vi "Main.vi"(11 "Module Admin":refnum<class "Delacor_lib_QMH_Module Admin.lvclass">) -> ()   [LabVIEW 2023, in "Adjust FP VIs.lvlib"]
doc: "This template is based off of the Queued Message Handler design pattern and the Queued Message Handler project template that ships with LabVIEW.\n\nThe main difference is that the queue is private to this module and communication between modules is performed via Broadcast and Request events.\n\nRequest events are wrapped in public API methods and are handled in the Event Handling Loop (EHL) of this VI. Any module can register for Broadcast events sent by this module. The EHL generates messages based on user interface actions.\n\nThe Message Handling Loop (MHL) processes messages generated by the EHL, or by other messages. The messages are string values, so new messages can be added easily to the Message Cases case structure in the MHL. Each message cluster can also provide an optional value for Message Data, which is a variant that can be converted to whatever message-specific data is required.\n_____\nBased on DQMH Dev Tools: Project Template 7.1.2.1547."
uses:
  Adjust FP VIs.lvlib
  <vilib>/Delacor/Delacor QMH/Libraries/Module Admin_class/Delacor_lib_QMH_Module Admin.lvclass
  Module Data--cluster.ctl
  Stop Argument--cluster.ctl
  <vilib>/Delacor/Delacor QMH/Libraries/Message Queue_class/Delacor_lib_QMH_Message Queue.lvclass/Delacor_lib_QMH_Message Queue.ctl
  <vilib>/Delacor/Delacor QMH/Libraries/Module Admin_class/Delacor_lib_QMH_Module Admin.lvclass/Delacor_lib_QMH_Module Admin.ctl
  <vilib>/Utility/miscctls.llb/LVPointTypeDef.ctl
  <vilib>/Delacor/Delacor QMH/Libraries/Message Queue_class/Delacor_lib_QMH_Enqueue Message (Single).vi
  <vilib>/Delacor/Delacor QMH/Libraries/Module Admin_class/Delacor_lib_QMH_Get External Launch.vi
  <vilib>/Delacor/Delacor QMH/Libraries/Message Queue_class/Delacor_lib_QMH_Message Queue.lvclass
  <resource>/dialog/QuickDrop/plugins/ZAlign/ZAlign.lvlib
panel:
  in  "OK Button":bool
  in  "Project Path":path
  out "Total VIs to Adjust":i32
  out "Front Panels Adjusted":u8(slide) scale=0.0..100.0
  out "error out":errorcluster
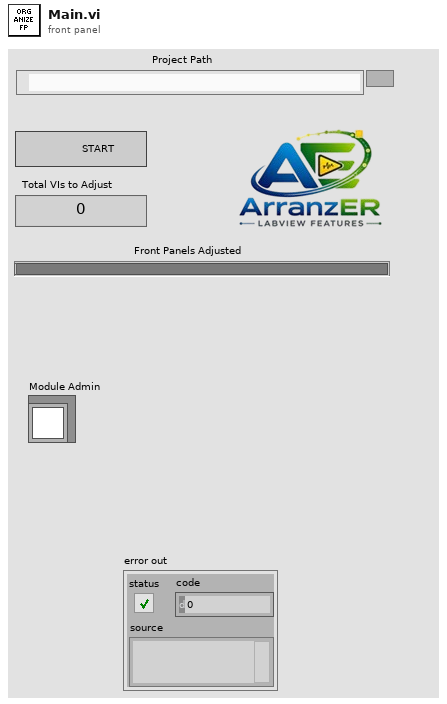
[diagram p1: front panel]
types:
  T1 = typedef "Adjust FP VIs.lvlib/Request Events--cluster.ctl" = cluster{"Stop Module":refnum<user-event>, "Show Panel":refnum<user-event>, "Hide Panel":refnum<user-event>, "Get Module Execution Status":refnum<user-event>, "Show Diagram":refnum<user-event>, "Private.Adjust FP for VIs":refnum<user-event>}
  T2 = typedef "Adjust FP VIs.lvlib/Module Data--cluster.ctl" = cluster{"Status":string, "VIs Name":string[], "VI Path List":path[], "Project Path":path, "Project:Open":refnum<vi>}
  T3 = typedef "LVPointTypeDef.ctl" = cluster{"Horizontal":i16, "Vertical":i16}
  T4 = enum32{"Invalid", "Standard", "Closed", "Hidden", "Minimized", "Maximized"}
  T5 = typedef "Adjust FP VIs.lvlib/Stop Argument--cluster.ctl" = cluster{"Origin":string, "Exit via Stop Module Req?":bool, "Wait for Module to stop?":bool}
  T6 = enum32{"invalid lock state", "Not Locked", "Locked (No Password)", "Password-protected"}
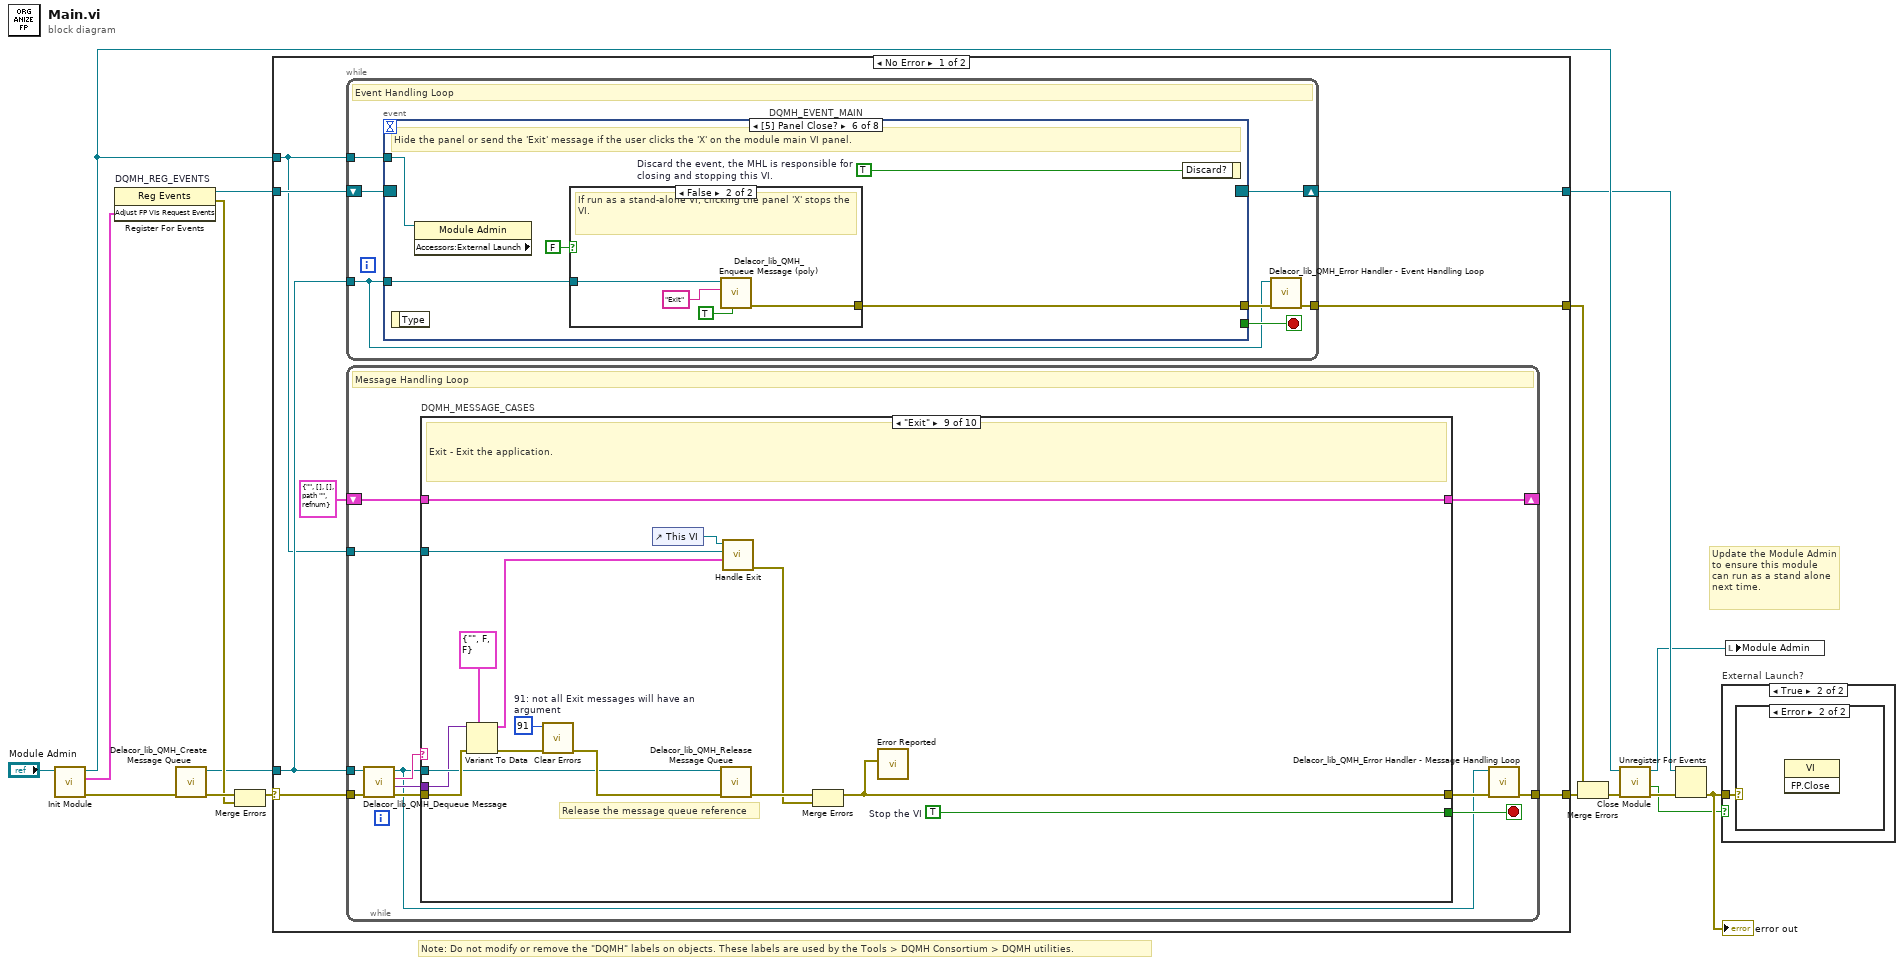
[diagram p0: block diagram]
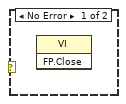
[diagram p3: hidden frame]
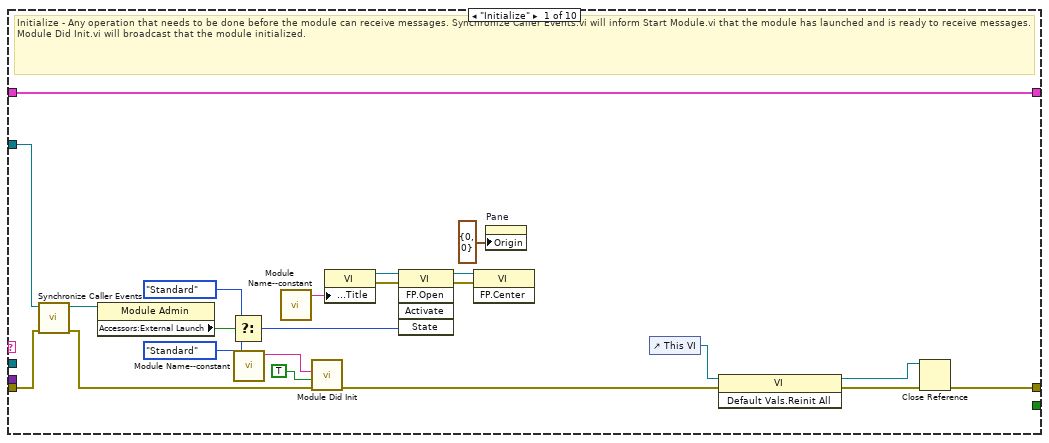
[diagram p4: hidden frame]
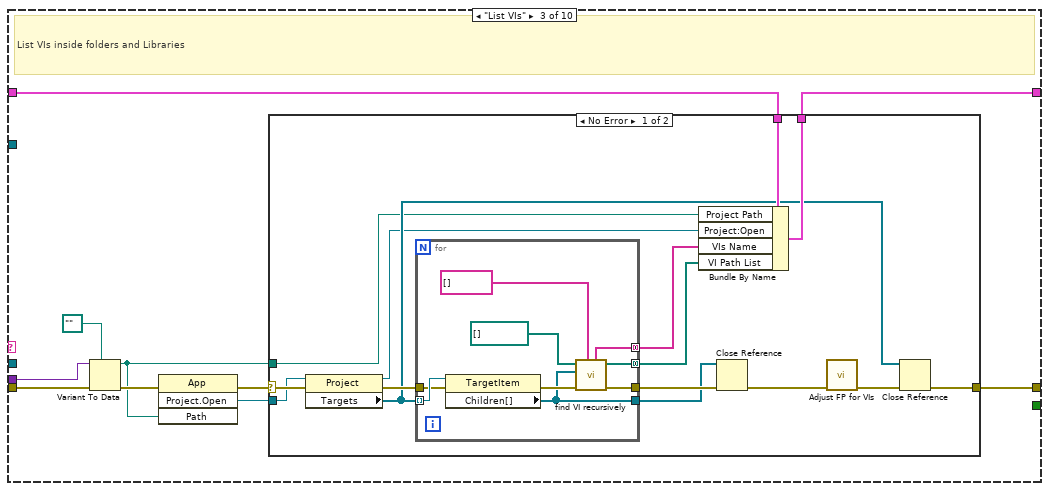
[diagram p6: hidden frame]
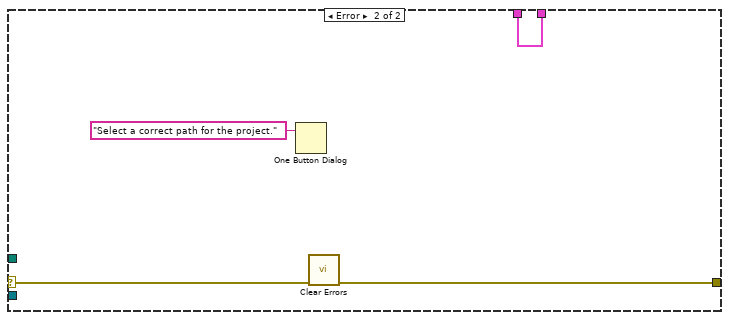
[diagram p7: hidden frame]
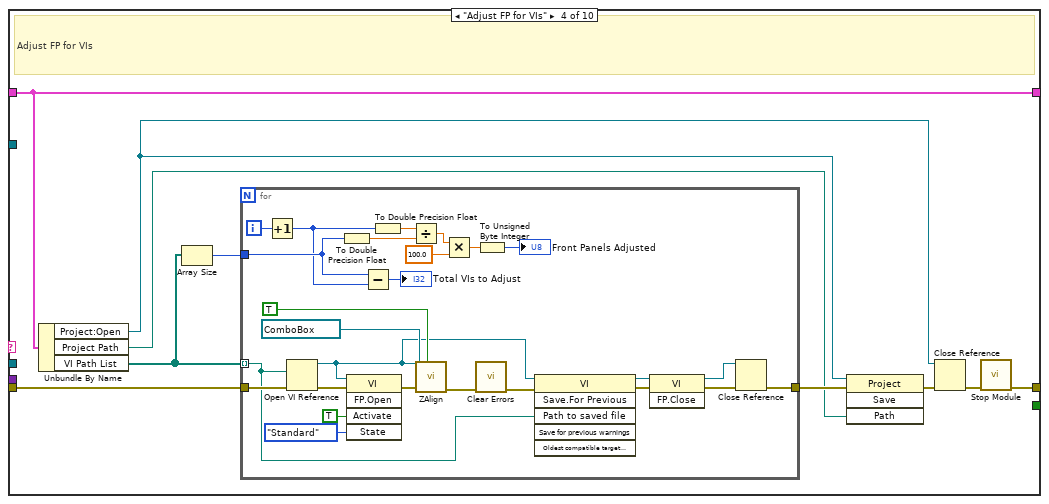
[diagram p8: hidden frame]
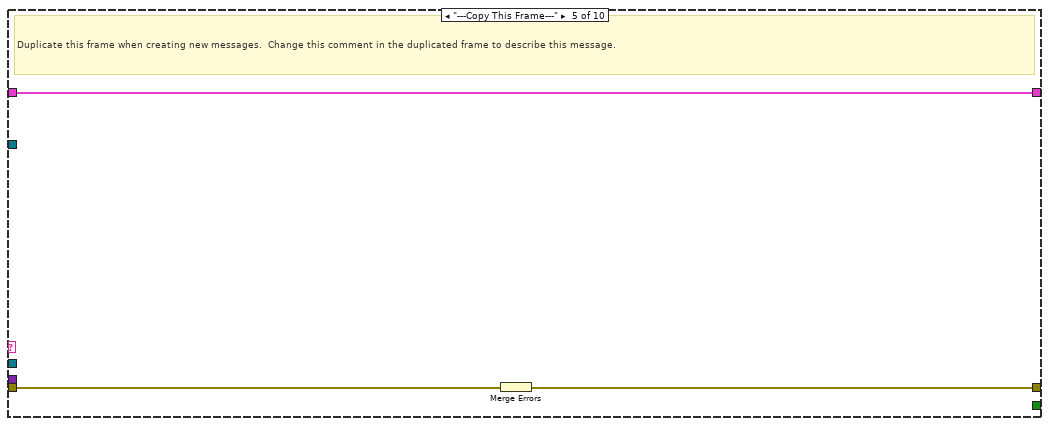
[diagram p9: hidden frame]
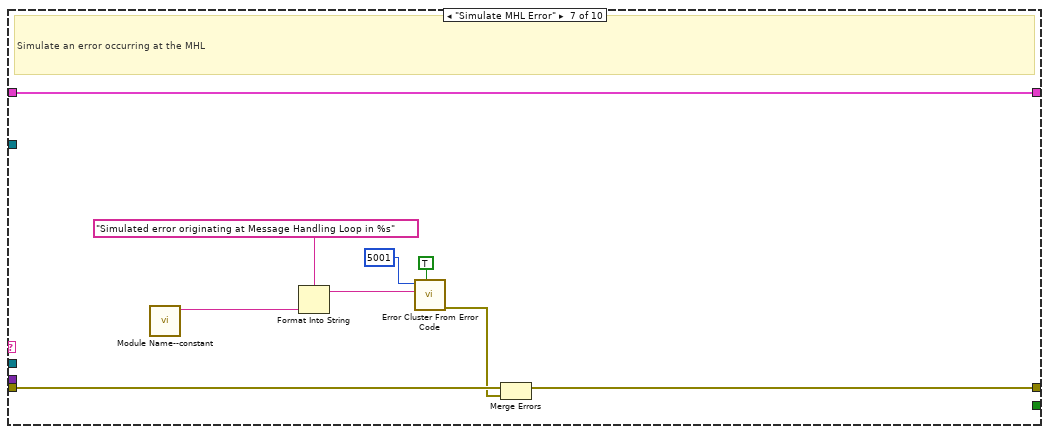
[diagram p11: hidden frame]
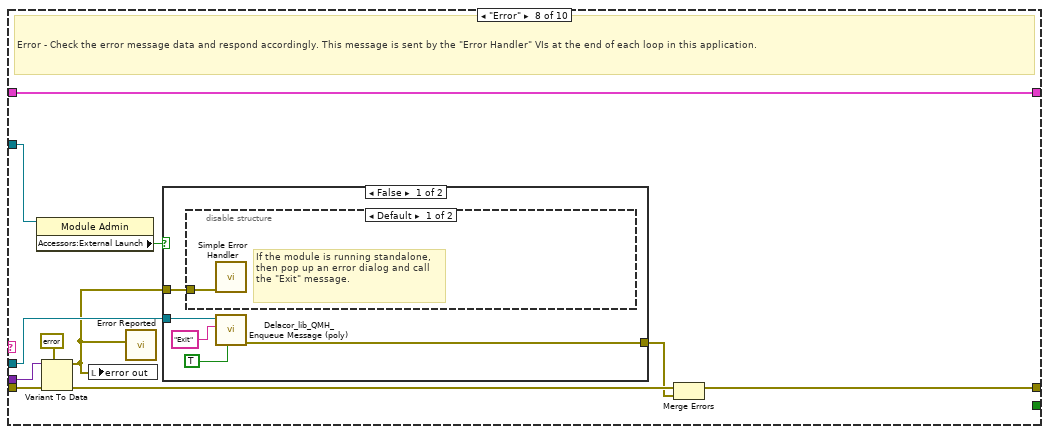
[diagram p12: hidden frame]
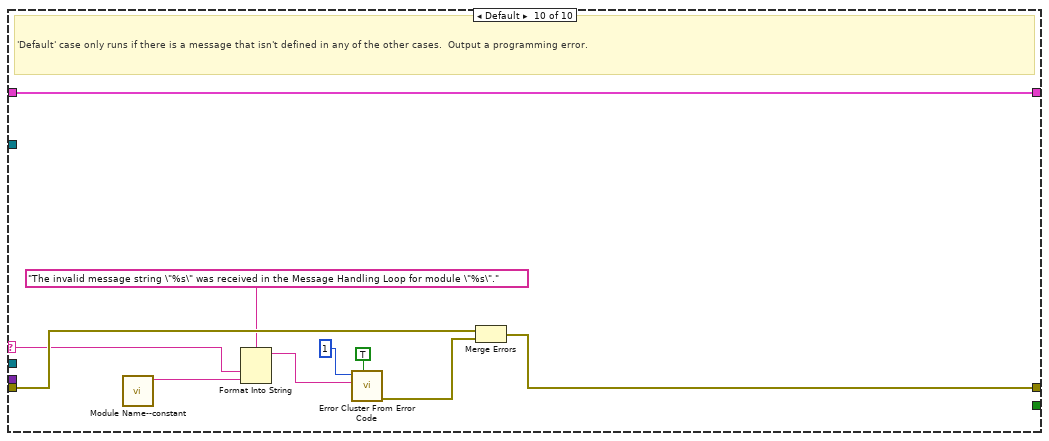
[diagram p15: hidden frame]
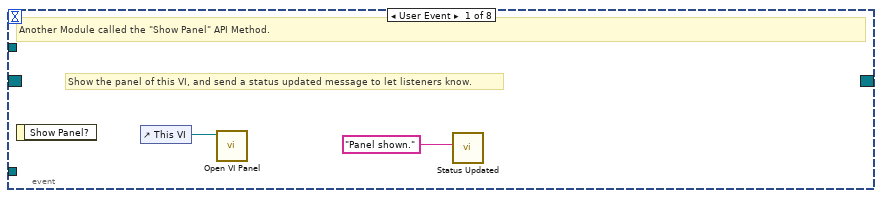
[diagram p16: hidden frame]
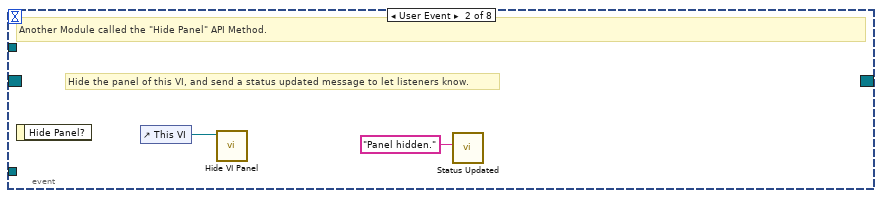
[diagram p17: hidden frame]
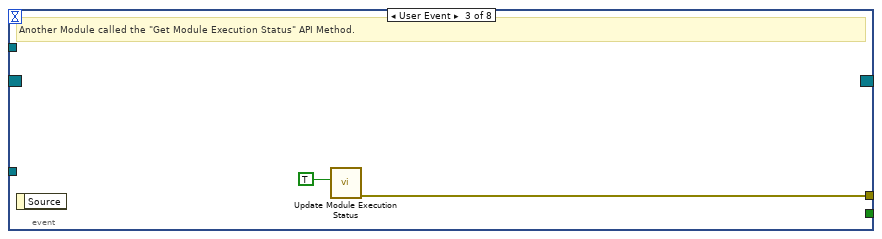
[diagram p18: hidden frame]
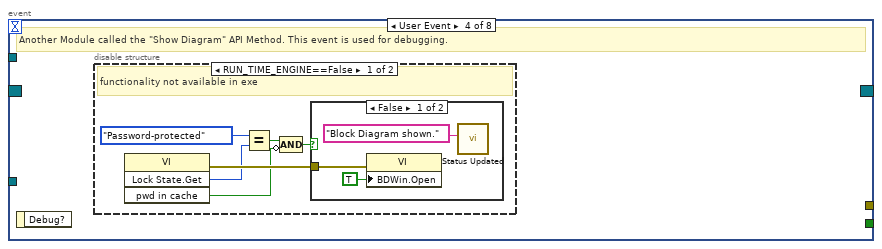
[diagram p19: hidden frame]
diagram:
  # "Note: Do not modify or remove the \"DQMH\" labels on objects. These labels are used by the Tools > DQMH Consortium > DQMH utilities."
  # "Update the Module Admin to ensure this module can run as a stand alone next time."
  n1 = call "Init Module.vi"("Singleton Module Admin in"="Module Admin") -> ("error out"=w16:errorcluster, "Adjust FP VIs Request Events"=w5:T1, "Singleton Module Admin out"=w8:refnum<class "Delacor_lib_QMH_Module Admin.lvclass">)  [unwired: 8 in]
  n2 = register-events "DQMH_REG_EVENTS"(w5) -> (reference out=w6:refnum<event-registration>, error out=w9:errorcluster)  [unwired: 2 in]
  n3 = call <vilib>:"Delacor_lib_QMH_Create Message Queue.vi"("error in"=w16) -> ("error out"=w11:errorcluster, "Message Queue"=w4:refnum<class "Delacor_lib_QMH_Message Queue.lvclass">)  [unwired: 9 in]
  n4 = Merge Errors(w11, w9) -> (w10:errorcluster)
  n5 = case shown="No Error" w10 {
    selector: w10 -> [w23 w251]
    tunnel: [w25 w250] -> w17
    tunnel: [w22 w249] -> w7
    tunnel: w6 -> [w20 w249]
    tunnel: w4 -> [w19 w244]
    tunnel: [w24 _] -> w14
    tunnel: w8 -> [w18 w245]
    frame No Error {
      n6 = while {
        tunnel: w19 -> [w192]
        shift-right: [w195] -> w22
        shift-left: w20 -> [w196]
        tunnel: [w197] -> w24
        tunnel: w18 -> [w193]
        stop <- w194 stop-if-true
        # "Event Handling Loop"
        n7 = event "DQMH_EVENT_MAIN" shown="[5] Panel Close?" {
          selector: w196 -> [_ _ _ _ _ _ _ _]
          dyn-events: [_ _ _ _ _ _ _ _] -> w195
          timeout: _ -> [_ _ _ _ _ _ _ _]
          tunnel: [_ _ _ _ TRUE ("Discard?") _ _ _] -> w194
          tunnel: w192 -> [_ _ _ _ w220 w227 w240 w243]
          tunnel: [_ _ w204 _ w223 w229 w238 w241] -> w198
          tunnel: w193 -> [_ _ _ _ _ w226 _ _]
          event User Event {
            # "Show the panel of this VI, and send a status updated message to let listeners know."
            # "Another Module called the \"Show Panel\" API Method."
            n8 = event-data() -> ()  [unwired: 1 in, 1 out]
            n9 = control-ref of="This VI"() -> (w200:refnum<vi>)
            n10 = call "Open VI Panel.vi"("VI"=w200) -> ()  [unwired: 10 in, 1 out]
            n11 = call "Status Updated.vi"("Status"="Panel shown." ("format string")) -> ()  [unwired: 10 in, 1 out]
          }
          event User Event {
            # "Hide the panel of this VI, and send a status updated message to let listeners know."
            # "Another Module called the \"Hide Panel\" API Method."
            n12 = event-data() -> ()  [unwired: 1 in, 1 out]
            n13 = control-ref of="This VI"() -> (w202:refnum<vi>)
            n14 = call "Hide VI Panel.vi"("VI"=w202) -> ()  [unwired: 10 in, 1 out]
            n15 = call "Status Updated.vi"("Status"="Panel hidden." ("format string")) -> ()  [unwired: 10 in, 1 out]
          }
          event User Event {
            # "Another Module called the \"Get Module Execution Status\" API Method."
            n16 = event-data() -> ()  [unwired: 1 in, 1 out]
            n17 = call "Update Module Execution Status.vi"("Running?"=TRUE) -> ("error out"=w204:errorcluster)  [unwired: 10 in]
          }
          event User Event {
            # "Another Module called the \"Show Diagram\" API Method. This event is used for debugging."
            n18 = event-data() -> ()  [unwired: 1 in, 1 out]
            n19 = disable-structure shown="RUN_TIME_ENGINE==False" {
              frame condition #0 (active) {
                # "functionality not available in exe"
                n20 = invoke on="Invoke Node" class="VI" method="Lock State.Get"() -> (error out=w210:errorcluster, "Get Lock State"=w209:T6, "pwd in cache"=w206:bool)  [unwired: 4 in, 1 out]
                n21 = Equal?(x=T6."Password-protected", y=w209) -> (x = y?=w207:bool)
                n22 = Compound Arithmetic op=AND(w207, invert w206) -> (w205:bool)
                n23 = case shown="False" w205 {
                  tunnel: w210 -> [w213 _]
                  frame False {
                    n24 = property on="Property Node" class="VI"(error in=w213, "BDWin.Open"=TRUE ("Block Diagram Window:Open")) -> ()  [unwired: 1 in, 2 out]
                    n25 = call "Status Updated.vi"("Status"="Block Diagram shown." ("format string")) -> ()  [unwired: 10 in, 1 out]
                  }
                  frame True {
                    # "Password-protected VI, and the password is not in the cache. Do not show the diagram."
                  }
                }
              }
              frame condition #1 {
              }
            }
          }
          event User Event {
            # "The Stop Module Event can get fired from the Exit message in the MHL. The queue gets destroyed in that case. If the queue no longer exists, the Enqueue Exit as a priority message will return error 1. It is safe to ignore, because the module is already exiting."
            # "Another Module called the \"Stop Module\" API Method  or the Message Handling Loop below."
            n26 = event-data() -> ("Exit via Stop Module Req?"=w216:bool, "Wait for Module to stop?"=w215:bool)  [unwired: 1 in]
            n27 = Bundle By Name(cluster=T5 {"Origin"="", "Exit via Stop Module Req?"=FALSE, "Wait for Module to stop?"=FALSE} ("Stop Argument"), "Exit via Stop Module Req?"=w216, "Wait for Module to stop?"=w215) -> (w214:T5)
            n28 = call-poly <vilib>:"Delacor_lib_QMH_Enqueue Message (poly).vi"("Priority Message? (F)"=TRUE, "Message Data"=w214, "Message"="Exit", "Message Queue in"=w220) -> ("error out"=w224:errorcluster)  [unwired: 6 in, 1 out]
            n29 = call <vilib>:"Clear Errors.vi"("error in (no error)"=w224, "specific error code to clear (0: all)"=1) -> ("error out"=w223:errorcluster)  [unwired: 4 in, 1 out]
          }
          event Panel Close? {
            w228 = TRUE  # Discard the event, the MHL is responsible for closing and stopping this VI.
            # "Hide the panel or send the 'Exit' message if the user clicks the 'X' on the module main VI panel."
            n30 = event-data() -> ()  [unwired: 1 in, 1 out]
            n31 = property on="Property Node" class="Module Admin" props=["Accessors:External Launch"](reference=w226) -> ()  [unwired: 1 in, 3 out]
            n32 = case shown="False" FALSE {
              tunnel: w227 -> [_ w235]
              tunnel: [_ w236] -> w229
              frame True {
                # "If externally launched, clicking the 'X' hides the panel, but doesn't close it."
                n33 = control-ref of="This VI"() -> (w232:refnum<vi>)
                n34 = call "Hide VI Panel.vi"("VI"=w232) -> ("error out"=w230:errorcluster)  [unwired: 10 in]
                n35 = call "Status Updated.vi"("error in"=w230, "Status"="Panel hidden." ("format string")) -> ()  [unwired: 9 in, 1 out]
              }
              frame False {
                # "If run as a stand-alone VI, clicking the panel 'X' stops the VI."
                n36 = call-poly <vilib>:"Delacor_lib_QMH_Enqueue Message (poly).vi"("Priority Message? (F)"=TRUE, "Message"="Exit", "Message Queue in"=w235) -> ("error out"=w236:errorcluster)  [unwired: 7 in, 1 out]
              }
            }
            n37 = event-data ("Event Filter Node")("Discard?"=w228) -> ()  [unwired: 1 in, 1 out]
          }
          event "OK Button": Value Change {
            # "This module called the \"Private.List VIs\" private request."
            n38 = event-data() -> ()  [unwired: 1 in, 1 out]
            n39 = call-poly <vilib>:"Delacor_lib_QMH_Enqueue Message (poly).vi"("Message Data"="Project Path", "Message"="List VIs", "Message Queue in"=w240) -> ("error out"=w238:errorcluster)  [unwired: 7 in, 1 out]
          }
          event User Event {
            # "This module called the \"Private.Adjust FP for VIs\" private request."
            n40 = event-data() -> ()  [unwired: 1 in, 1 out]
            n41 = call-poly <vilib>:"Delacor_lib_QMH_Enqueue Message (poly).vi"("Message"="Adjust FP for VIs", "Message Queue in"=w243) -> ("error out"=w241:errorcluster)  [unwired: 8 in, 1 out]
          }
        }
        n42 = call-dynamic "Delacor_lib_QMH_Error Handler - Event Handling Loop.vi"("error in"=w198, "Message Queue in"=w192) -> ("dup error in"=w197:errorcluster)  [unwired: 8 in, 1 out]
      }
      n43 = while {
        tunnel: w19 -> [w26]
        shift-right: [w34] -> _
        shift-left: T2 {"Status"="", "VIs Name"=[], "VI Path List"=[], "Project Path"=path "", "Project:Open"=refnum} ("Data Cluster") -> [w35]
        tunnel: w23 -> [w37]
        tunnel: [w29] -> w25
        tunnel: w18 -> [w30]
        stop <- w33 stop-if-true
        # "Message Handling Loop"
        n44 = call-dynamic "Delacor_lib_QMH_Dequeue Message.vi"("error in"=w37, "Message Queue in"=w26) -> ("error out"=w36:errorcluster, "Message Data"=w31:variant, "Message"=w32:string, "Message Queue out"=w27:refnum<class "Delacor_lib_QMH_Message Queue.lvclass">)  [unwired: 6 in]
        n45 = case "DQMH_MESSAGE_CASES" shown="\"Exit\"" w32 {
          selector: w32 -> [_ _ _ _ _ _ _ _ _ w187]
          tunnel: w27 -> [_ _ _ _ _ _ _ w153 w175 _]
          tunnel: w36 -> [w57 w61 w68 w109 w138 w140 w149 w160 w181 w190]
          tunnel: [w40 w61 w69 w102 w137 w140 w148 w156 w176 w191] -> w28
          tunnel: w35 -> [w47 w60 w70 w108 w136 w139 w146 w155 w167 w188]
          tunnel: [w47 w60 w71 w108 w136 w139 w146 w155 w167 w188] -> w34
          tunnel: [_ _ _ _ _ _ _ _ w174 _] -> w33
          tunnel: w31 -> [_ _ w63 _ _ _ _ w154 w173 _]
          tunnel: w30 -> [w48 _ _ _ _ _ _ w152 w168 _]
          frame "Initialize" {
            # "Initialize - Any operation that needs to be done before the module can receive messages. Synchronize Caller Events.vi will inform Start Module.vi that the module has launched and is ready to receive messages. Module Did Init.vi will broadcast that the module initialized."
            n46 = call "Synchronize Caller Events.vi"("error in"=w57, "Singleton Module Admin in"=w48) -> ("error out"=w56:errorcluster, "Singleton Module Admin out"=w44:refnum<class "Delacor_lib_QMH_Module Admin.lvclass">)  [unwired: 8 in]
            n47 = property on="Property Node" class="Module Admin"(reference=w44) -> ("Accessors:External Launch"=w52:bool)  [unwired: 1 in, 2 out]
            n48 = Select(t=T4."Standard" ("State"), s=w52, f=T4."Standard" ("State")) -> (s? t:f=w49:T4)
            n49 = call "Module Name--constant.vi"() -> ("Module Name"=w45:string)  [unwired: 11 in]
            n50 = call "Module Name--constant.vi"() -> ("Module Name"=w55:string)  [unwired: 11 in]
            n51 = call "Module Did Init.vi"("error in"=w56, "Initialized?"=TRUE, "Origin"=w45) -> ("error out"=w38:errorcluster)  [unwired: 8 in]
            n52 = property on="Property Node" class="VI"("Front Panel.Title"=w55) -> (reference out=w54:refnum<vi>, error out=w59:errorcluster)  [unwired: 2 in]
            n53 = invoke on="Invoke Node" class="VI" method="FP.Open"(reference=w54, error in=w59, "State"=w49) -> (reference out=w53:refnum<vi>, error out=w58:errorcluster)  [unwired: 2 in, 3 out]
            n54 = invoke on="Invoke Node" class="VI" method="FP.Center"(reference=w53, error in=w58) -> ()  [unwired: 1 in, 3 out]
            n55 = property on="Pane" class="Pane"("Origin"=T3 {"Horizontal"=0, "Vertical"=0}) -> ()  [unwired: 2 in, 2 out]
            n56 = control-ref of="This VI"() -> (w41:refnum<vi>)
            n57 = invoke class="VI" method="Default Vals.Reinit All"(reference=w41, error in=w38) -> (reference out=w39:refnum<vi>, error out=w42:errorcluster)  [unwired: 1 in, 1 out]
            n58 = Close Reference(reference=w39, error in (no error)=w42) -> (error out=w40:errorcluster)
          }
          frame "---Module Specific---" {
            # "Separator -- The following cases handle messages specific to this Module."
          }
          frame "List VIs" {
            # "List VIs inside folders and Libraries"
            n59 = Variant To Data(error in=w68, type=path "", Variant=w63) -> (data=w62:path, error out=w65:errorcluster)
            n60 = invoke class="App" method="Project.Open"(error in=w65, "Path"=w62) -> (error out=w66:errorcluster, "Project:Open"=w67:refnum<vi>)  [unwired: 2 in, 2 out]
            n61 = case shown="No Error" w66 {
              selector: w66 -> [w79 w99]
              tunnel: [w83 w98] -> w71
              tunnel: w70 -> [w82 w98]
              tunnel: [w78 w96] -> w69
              tunnel: w67 -> [w76 _]
              tunnel: w62 -> [w75 _]
              frame No Error {
                n62 = property on="Property Node" class="Project"(reference=w76, error in=w79) -> (reference out=w74:refnum<vi>, error out=w86:errorcluster, "Targets"=w77:refnum<vi>[])
                n63 = for {
                  tunnel: w77 -> [w95] mode=indexing
                  tunnel: w86 -> [w94]
                  tunnel: [w90] -> w81
                  tunnel: [w89] -> w84 mode=concatenating
                  tunnel: [w88] -> w85 mode=concatenating
                  tunnel: [w87] -> w72
                  n64 = property on="Property Node" class="TargetItem"(reference=w95, error in=w94) -> (error out=w92:errorcluster, "Children[]"=w87:refnum<vi>[])  [unwired: 1 out]
                  n65 = call "find VI recursively.vi"("VIs Name"=string[] [], "error in (no error)"=w92, "Project Item"=w87, "VI Ref In"=path[] [] ("Array")) -> ("error out"=w90:errorcluster, "VI Ref Out"=w89:path[], "VIs Name Out"=w88:string[])  [unwired: 5 in]
                }
                n66 = Bundle By Name(cluster=w82, "Project Path"=w75, "Project:Open"=w74, "VIs Name"=w85, "VI Path List"=w84) -> (w83:T2)
                n67 = Close Reference(reference=w72, error in (no error)=w81) -> (error out=w73:errorcluster)
                n68 = call "Adjust FP for VIs.vi"("error in"=w73) -> ("error out"=w80:errorcluster)  [unwired: 10 in]
                n69 = Close Reference(reference=w77, error in (no error)=w80) -> (error out=w78:errorcluster)
              }
              frame Error {
                n70 = One Button Dialog(message="Select a correct path for the project.") -> ()  [unwired: 1 in, 1 out]
                n71 = call <vilib>:"Clear Errors.vi"("error in (no error)"=w99) -> ("error out"=w96:errorcluster)  [unwired: 5 in, 1 out]
              }
            }
          }
          frame "Adjust FP for VIs" {
            # "Adjust FP for VIs"
            n72 = Unbundle By Name(w108) -> ("Project:Open"=w104:refnum<vi>, "Project Path"=w105:path, "VI Path List"=w100:path[])
            n73 = Array Size(array=w100) -> (size(s)=w107:i32)
            n74 = for {
              tunnel: w109 -> [w124]
              tunnel: [w123] -> w106
              tunnel: w107 -> [w126]
              tunnel: w100 -> [w122] mode=indexing
              i -> [w135]
              n75 = Increment(x=w135) -> (x+1=w125:i32)
              n76 = Open VI Reference(vi path=w122, error in (no error)=w124) -> (vi reference=w118:refnum<vi>, error out=w128:errorcluster)  [unwired: 4 in]
              n77 = To Double Precision Float(number=w126) -> (double precision float=w133:dbl)
              n78 = invoke class="VI" method="FP.Open"(reference=w118, error in=w128, "Activate"=TRUE ("Activate?"), "State"=T4."Standard") -> (error out=w112:errorcluster)  [unwired: 1 in, 4 out]
              n79 = Subtract(x=w126, y=w125) -> (x-y=→"Total VIs to Adjust":i32)
              n80 = To Double Precision Float(number=w125) -> (double precision float=w134:dbl)
              n81 = Divide(x=w134, y=w133) -> (x/y=w132:dbl)
              n82 = call <resource>:"ZAlign.vi"("Shift Pressed?"=TRUE, "error in (no error)"=w112, "QD Combo Box Ref"=refnum<vi> refnum, "QD Launch VI Ref"=w118) -> ("error out"=w111:errorcluster)  [unwired: 6 in, 1 out]
              n83 = Multiply(x=w132, y=100.0) -> (x*y=w130:dbl)
              n84 = call <vilib>:"Clear Errors.vi"("error in (no error)"=w111) -> ("error out"=w110:errorcluster)  [unwired: 5 in, 1 out]
              n85 = To Unsigned Byte Integer(number=w130) -> (unsigned 8bit integer=→"Front Panels Adjusted":u8)
              n86 = invoke class="VI" method="Save.For Previous"(reference=w118, error in=w110, "Path to saved file"=w122) -> (reference out=w114:refnum<vi>, error out=w119:errorcluster)  [unwired: 3 in, 4 out]
              n87 = invoke class="VI" method="FP.Close"(reference=w114, error in=w119) -> (reference out=w113:refnum<vi>, error out=w115:errorcluster)  [unwired: 1 in, 1 out]
              n88 = Close Reference(reference=w113, error in (no error)=w115) -> (error out=w123:errorcluster)
            }
            n89 = invoke class="Project" method="Save"(reference=w104, error in=w106, "Path"=w105) -> (error out=w101:errorcluster)  [unwired: 1 in, 3 out]
            n90 = Close Reference(reference=w104, error in (no error)=w101) -> (error out=w103:errorcluster)
            n91 = call "Stop Module.vi"("error in"=w103) -> ("error out"=w102:errorcluster)  [unwired: 10 in]
          }
          frame "---Copy This Frame---" {
            # "Duplicate this frame when creating new messages.  Change this comment in the duplicated frame to describe this message."
            n92 = Merge Errors(w138) -> (w137:errorcluster)
          }
          frame "---Exit and Error Handling---" {
            # "Separator - The following cases handle errors and exit messages."
          }
          frame "Simulate MHL Error" {
            # "Simulate an error occurring at the MHL"
            n93 = call "Module Name--constant.vi"() -> ("Module Name"=w142:string)  [unwired: 11 in]
            n94 = Format Into String(format string="Simulated error originating at Message Handling Loop in %s", w142) -> (resulting string=w143:string)  [unwired: 2 in, 1 out]
            n95 = call <vilib>:"Error Cluster From Error Code.vi"("show call chain? (False)"=TRUE, "error message (\"\")"=w143, "error code (0)"=5001) -> ("error out"=w147:errorcluster)  [unwired: 6 in]
            n96 = Merge Errors(w149, w147) -> (w148:errorcluster)
          }
          frame "Error" {
            # "Error - Check the error message data and respond accordingly. This message is sent by the \"Error Handler\" VIs at the end of each loop in this application."
            n97 = property on="Property Node" class="Module Admin"(reference=w152) -> ("Accessors:External Launch"=w151:bool)  [unwired: 1 in, 2 out]
            n98 = Variant To Data(error in=w160, type=errorcluster {"status"=FALSE, "code"=0, "source"=""} ("error constant"), Variant=w154) -> (data=w150:errorcluster, error out=w158:errorcluster)
            n99 = local write "error out"(w150) -> ()
            n100 = call "Error Reported.vi"("Error"=w150) -> ()  [unwired: 10 in, 1 out]
            n101 = case shown="False" w151 {
              tunnel: [w165 _] -> w157
              tunnel: w153 -> [w163 _]
              tunnel: w150 -> [w164 _]
              frame False {
                n102 = disable-structure shown="Default" {
                  disable-tunnel: w164 -> [w166 _]
                  frame condition #0 (active) {
                    # "If the module is running standalone, then pop up an error dialog and call the \"Exit\" message."
                    n103 = call <vilib>:"Simple Error Handler.vi"("error in (no error)"=w166) -> ()  [unwired: 4 in, 5 out]
                  }
                  frame condition #1 {
                    # "To prevent the Simple Error Handler VI from being loaded (e.g. when deploying to a Real-Time target), add the Conditional Disable Symbol \"DQMH_Disable_SEH\" to your project and set it to TRUE."
                  }
                }
                n104 = call-poly <vilib>:"Delacor_lib_QMH_Enqueue Message (poly).vi"("Priority Message? (F)"=TRUE, "Message"="Exit", "Message Queue in"=w163) -> ("error out"=w165:errorcluster)  [unwired: 7 in, 1 out]
              }
              frame True {
                # "If the module was launched externally, calling the Error Reported broadcast VI is the only action performed by the \"Error\" message. The module's caller can then process the error appropriately."
              }
            }
            n105 = Merge Errors(w158, w157) -> (w156:errorcluster)
          }
          frame "Exit" {
            w172 = 91  # 91: not all Exit messages will have an argument
            w174 = TRUE  # Stop the VI
            # "Release the message queue reference"
            # "Exit - Exit the application."
            n106 = Variant To Data(error in=w181, type=T5 {"Origin"="", "Exit via Stop Module Req?"=FALSE, "Wait for Module to stop?"=FALSE} ("Stop Argument"), Variant=w173) -> (data=w170:T5, error out=w178:errorcluster)
            n107 = call <vilib>:"Clear Errors.vi"("error in (no error)"=w178, "specific error code to clear (0: all)"=w172) -> ("error out"=w180:errorcluster)  [unwired: 4 in, 1 out]
            n108 = control-ref of="This VI"() -> (w169:refnum<vi>)
            n109 = call-dynamic "Delacor_lib_QMH_Release Message Queue.vi"("error in"=w180, "Message Queue"=w175) -> ("error out"=w179:errorcluster)  [unwired: 9 in]
            n110 = call "Handle Exit.vi"("Stop Argument"=w170, "Admin in"=w168, "VI reference"=w169) -> ("error out"=w177:errorcluster)  [unwired: 7 in, 1 out]
            n111 = Merge Errors(w179, w177) -> (w176:errorcluster)
            n112 = call "Error Reported.vi"("Error"=w176) -> ()  [unwired: 10 in, 1 out]
          }
          frame Default {
            # "'Default' case only runs if there is a message that isn't defined in any of the other cases.  Output a programming error."
            n113 = call "Module Name--constant.vi"() -> ("Module Name"=w186:string)  [unwired: 11 in]
            n114 = Format Into String(format string="The invalid message string \"%s\" was received in the Message Handling Loop for module \"%s\".", w187, w186) -> (resulting string=w182:string)  [unwired: 2 in, 1 out]
            n115 = call <vilib>:"Error Cluster From Error Code.vi"("show call chain? (False)"=TRUE, "error message (\"\")"=w182, "error code (0)"=1) -> ("error out"=w189:errorcluster)  [unwired: 6 in]
            n116 = Merge Errors(w190, w189) -> (w191:errorcluster)
          }
        }
        n117 = call-dynamic "Delacor_lib_QMH_Error Handler - Message Handling Loop.vi"("error in"=w28, "Message Queue in"=w27) -> ("dup error in"=w29:errorcluster)  [unwired: 8 in, 1 out]
      }
    }
    frame Error {
      # "Synchronize Caller Events.vi will inform Start Module.vi that the module has launched and will let the code calling Start Module.vi register for broadcasts and would permit the caller receive the broadcast that an error occurred at launch time."
      n118 = call-dynamic "Delacor_lib_QMH_Release Message Queue.vi"("error in"=w251, "Message Queue"=w244) -> ("error out"=w250:errorcluster)  [unwired: 9 in]
      n119 = call "Synchronize Caller Events.vi"("Singleton Module Admin in"=w245) -> ("error out"=w252:errorcluster)  [unwired: 9 in, 1 out]
      n120 = call "Module Name--constant.vi"() -> ("Module Name"=w248:string)  [unwired: 11 in]
      n121 = Format Into String(format string="An error occurred during initialization. %s is no longer running.", w248) -> (resulting string=w246:string)  [unwired: 2 in, 1 out]
      n122 = Merge Errors(w250, w252) -> (w253:errorcluster)
      n123 = call "Error Reported.vi"("Additional Information"=w246, "Error"=w253) -> ()  [unwired: 9 in, 1 out]
    }
  }
  n124 = Merge Errors(w14, w17) -> (w13:errorcluster)
  n125 = call "Close Module.vi"("error in"=w13, "Module Admin in"=w8) -> ("error out"=w15:errorcluster, "External Launch"=w1:bool, "Module Admin out"=w2:refnum<class "Delacor_lib_QMH_Module Admin.lvclass">)  [unwired: 7 in]
  n126 = Unregister For Events(event registration refnum=w7, error in=w15) -> (error out=w12:errorcluster)
  "error out" <- w12
  n127 = case "External Launch?" shown="True" w1 {
    tunnel: w12 -> [_ w254]
    frame False {
    }
    frame True {
      n128 = case shown="Error" w254 {
        frame No Error {
          n129 = invoke on="Invoke Node" class="VI" method="FP.Close"() -> ()  [unwired: 3 in, 3 out]
        }
        frame Error {
          n130 = invoke on="Invoke Node" class="VI" method="FP.Close"() -> ()  [unwired: 3 in, 3 out]
        }
      }
    }
  }
  n131 = local write "Module Admin"(w2) -> ()
